vi "FV_motor_end.vi"(8 "error in (no error)":errorcluster, 11 "VISA Refnum in":refnum<visa-resource-name>) -> (0 "error out":errorcluster)   [LabVIEW 2019]
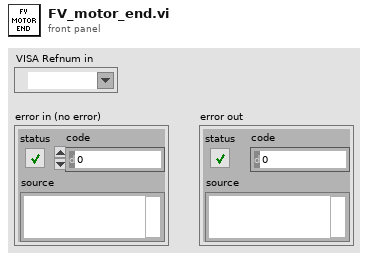
[diagram p1: front panel]
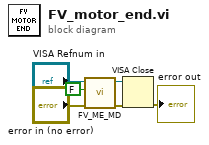
[diagram p0: block diagram]
diagram:
  n1 = call "FV_ME_MD.vi"("error in"="error in (no error)", "enable_or_disable"=FALSE, "VISA in"="VISA Refnum in") -> ("error out"=w5:errorcluster, "VISA out"=w3:refnum<visa-resource-name>)  [unwired: 6 in, 1 out]
  n2 = VISA Close(VISA resource name=w3, error in (no error)=w5) -> (error out=→"error out":errorcluster)
